vi "scan_discovery.vi"() -> (3 "module configuration out":refnum<class "Scan Engine configuration.lvclass">)   [LabVIEW 2013]
uses:
  configuration/Scan Engine configuration.lvclass
  execution/Scan Engine runtime.lvclass
  <vilib>/NI/TBM Modules/iov/module/configuration/Scan Engine configuration.lvclass
  <vilib>/NI/Tag Bus Module Framework/channel/TBM channel.lvclass
panel:
  out "error out":errorcluster
  out "All Channels":string
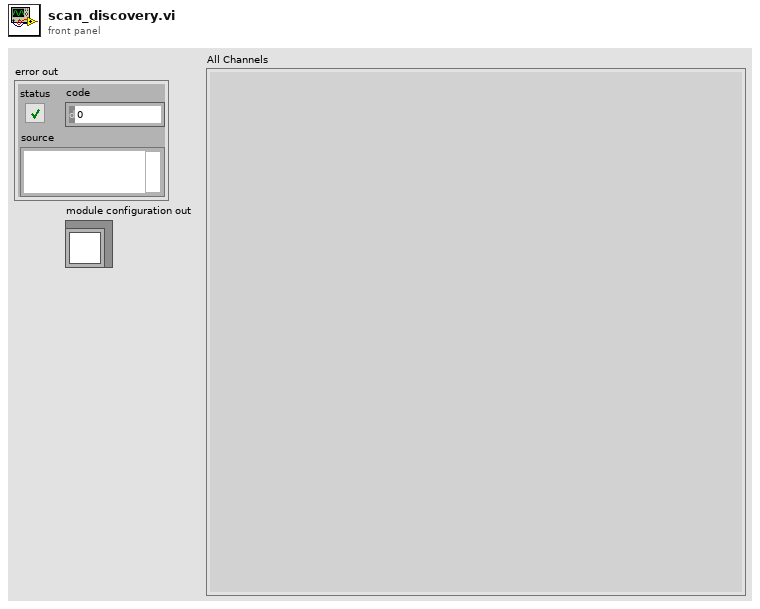
[diagram p1: front panel]
types:
  T1 = typedef "tag bus.lvlib/tag descriptor.lvclass/Data Type.ctl" = enum16{"Double", "Single", "I64", "I32", "I16", "I8", "U64", "U32", "U16", "U8", "Boolean", "String", "Array of Double", "Array of Single", "Array of I64", "Array of I32", "Array of I16", "Array of I8", "Array of U64", "Array of U32", "Array of U16", "Array of U8", "Array of Boolean", "Array of String"}
  T2 = typedef "TBM channel.lvclass/channel classification.ctl" = enum16{"input data", "output data", "processing parameter", "processing result"}
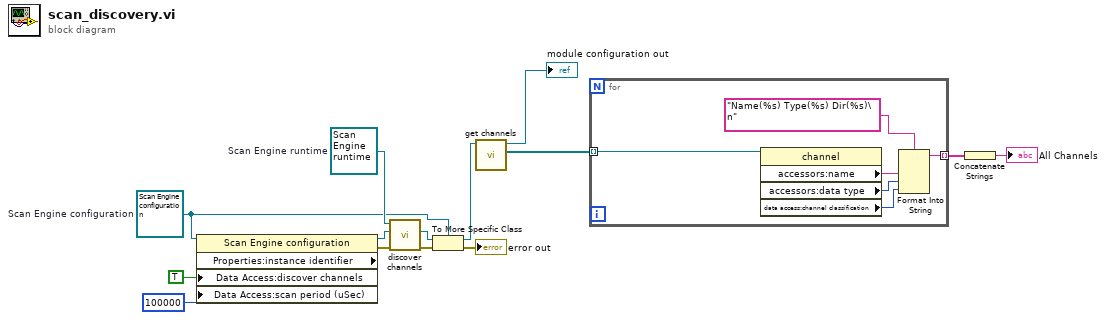
[diagram p0: block diagram]
diagram:
  w12 = refnum<class "Scan Engine runtime.lvclass"> refnum  # Scan Engine runtime
  w9 = refnum<class "Scan Engine configuration.lvclass"> refnum  # Scan Engine configuration
  n1 = property class="Scan Engine configuration" props=["Properties:instance identifier", "Data Access:discover channels", "Data Access:scan period (uSec)"](reference=w9, "Data Access:discover channels"=TRUE ("discover channels"), "Data Access:scan period (uSec)"=u32 100000 ("scan period (uSec)")) -> (reference out=w11:refnum<class "Scan Engine configuration.lvclass">, error out=w3:errorcluster)  [unwired: 1 in, 1 out]
  n2 = call-dynamic "discover channels.vi"("error in"=w3, "module configuration"=w11, "module in"=w12) -> ("error out"=w2:errorcluster, "updated configuration"=w10:refnum<class "TBM module configuration.lvclass">)  [unwired: 6 in, 1 out]
  n3 = To More Specific Class(target class=w9, reference=w10, error in=w2) -> (specific class reference=w8:refnum<class "Scan Engine configuration.lvclass">, error out=→"error out":errorcluster)
  n4 = call-dynamic "get channels.vi"("module configuration in"=w8) -> ("channels"=w7:refnum<class "TBM channel.lvclass">[], "module configuration out"=→"module configuration out":refnum<class "Scan Engine configuration.lvclass">)  [unwired: 9 in]
  n5 = for {
    tunnel: w7 -> [w20] mode=indexing
    tunnel: [w15] -> w6 mode=indexing
    n6 = property class="channel"(reference=w20) -> ("accessors:name"=w19:string, "accessors:data type"=w18:T1, "data access:channel classification"=w17:T2)  [unwired: 1 in, 2 out]
    n7 = Format Into String(format string="Name(%s) Type(%s) Dir(%s)\n", w19, w18, w17) -> (resulting string=w15:string)  [unwired: 2 in, 1 out]
  }
  n8 = Concatenate Strings(w6) -> (→"All Channels":string)
